vi "Command_Follow_Path.vi"(7 "Startup":bool, 8 "timeout":dbl, 9 "acceptable angle error":dbl, 10 "acceptable distance error":dbl, 11 "file_name":string) -> (1 "Turn Speed(rad/s)":dbl, 2 "Linear Speed(in/s)":dbl, 4 "Reint":bool, 6 "Completed":bool)   [LabVIEW 2019]
uses:
  Auto Utilities/Command_Execution_State.ctl
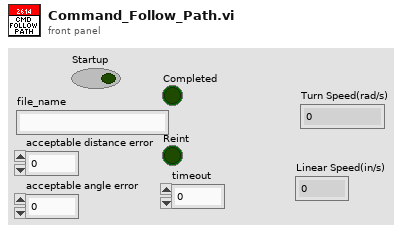
[diagram p1: front panel]
types:
  T1 = typedef "Command_Execution_State.ctl" = enum16{"Initialize", "Execute", "Finish"}
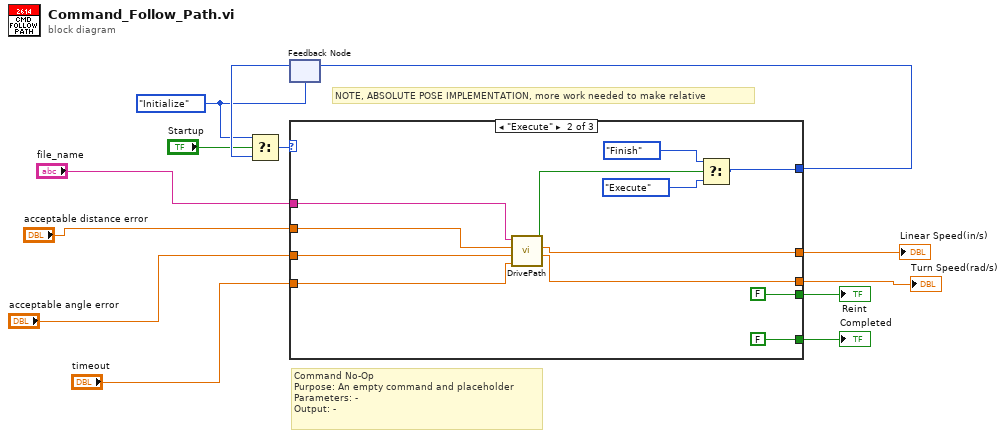
[diagram p0: block diagram]
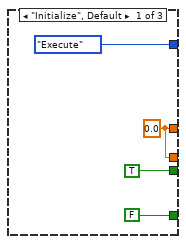
[diagram p2: hidden frame]
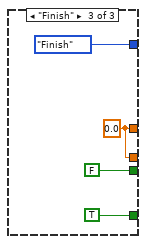
[diagram p3: hidden frame]
diagram:
  w7 = Command_Execution_State."Initialize" ("Play State")
  # "NOTE, ABSOLUTE POSE IMPLEMENTATION, more work needed to make relative"
  # "Command No-Op\nPurpose: An empty command and placeholder\nParameters: -\nOutput: -"
  n1 = feedback #1(w7) -> (w11:T1)
  n2 = Select(t=w7, s="Startup", f=w11) -> (s? t:f=w13:T1)
  n3 = case shown="\"Execute\"" w13 {
    tunnel: [Command_Execution_State."Execute" ("Play State") w21 Command_Execution_State."Finish" ("Play State")] -> w12
    tunnel: [FALSE FALSE TRUE] -> w10
    tunnel: [TRUE FALSE FALSE] -> w8
    tunnel: "file_name" -> [_ w27 _]
    tunnel: "acceptable distance error" -> [_ w26 _]
    tunnel: "acceptable angle error" -> [_ w25 _]
    tunnel: "timeout" -> [_ w24 _]
    tunnel: [w14 w23 w30] -> w2
    tunnel: [w14 w22 w30] -> w1
    frame "Initialize", Default {
      w14 = 0.0 ("Linear Speed(in/s)")
    }
    frame "Execute" {
      n4 = call "DrivePath.vi"("timeout"=w24, "acceptable angle error"=w25, "acceptable distance error"=w26, "file_name"=w27) -> ("Turn Speed(rad/s)"=w22:dbl, "Linear Speed(in/s)"=w23:dbl, "Finish?"=w18:bool)  [unwired: 5 in]
      n5 = Select(t=Command_Execution_State."Finish" ("Play State"), s=w18, f=Command_Execution_State."Execute" ("Play State")) -> (s? t:f=w21:T1)
    }
    frame "Finish" {
      w30 = 0.0 ("Linear Speed(in/s)")
    }
  }
  "Completed" <- w10
  "Reint" <- w8
  "Linear Speed(in/s)" <- w2
  "Turn Speed(rad/s)" <- w1
  n6 = feedback-in #1(w12) -> ()
